vi "saveFile(subVI).vi"(1 "Typ signálu":string, 2 "Vstupní signál":waveform(dbl)) -> ()   [LabVIEW 2026]
uses:
  <vilib>/Utility/file.llb/Write Delimited Spreadsheet (DBL).vi
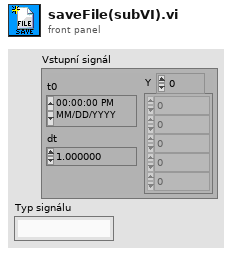
[diagram p1: front panel]
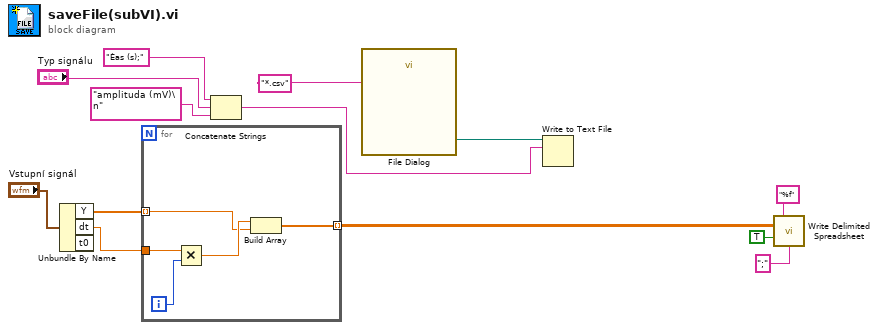
[diagram p0: block diagram]
diagram:
  n1 = Unbundle By Name("Vstupní signál") -> ("Y"=w12:dbl[], "dt"=w11:dbl)  [unwired: 1 out]
  n2 = for {
    tunnel: w12 -> [w15] mode=indexing
    tunnel: w11 -> [w17]
    tunnel: [w14] -> w10 mode=indexing
    i -> [w18]
    n3 = Multiply(x=w17, y=w18) -> (x*y=w16:dbl)
    n4 = Build Array(w16, w15) -> (w14:dbl[])
  }
  n5 = Concatenate Strings("Èas (s);", "Typ signálu", "amplituda (mV)\n") -> (w2:string)
  n6 = call "File Dialog"("pattern (all files)"="*.csv") -> ("selected path"=w6:path)  [unwired: 11 in, 3 out]
  n7 = Write to Text File(file (use dialog)=w6, text=w2) -> ()  [unwired: 2 in, 3 out]
  n8 = call-poly <vilib>:"Write Delimited Spreadsheet.vi"("format (%.3f)"="%f", "2D data"=w10, "append to file? (new file:F)"=TRUE, "delimiter (\\t)"=";" ("delimiter (\\t)")) -> ()  [unwired: 10 in, 2 out]
